vi "Get Records by Channels.vi"(6 "Channel List (All)":string, 8 "error in (no error)":errorcluster, 9 "Record Length (-1)":i32=-1, 10 "Record Start Index (0)":i32, 11 "Live Graph Plotter in":refnum<class "Live Graph Plotter.lvclass">) -> (0 "error out":errorcluster, 2 "Records By Channels":T1(array[cluster]), 3 "Live Graph Plotter out":refnum<class "Live Graph Plotter.lvclass">, 4 "Channel List":string)   [LabVIEW 2025, in "Live Graph Plotter.lvclass"]
uses:
  Live Graph Plotter.lvclass
  Live Graph Plotter.lvclass/Live Graph Plotter.ctl
  <vilib>/regexp/Match Regular Expression.xnode
  <vilib>/Analysis/NI_AALBase.lvlib
  26139874-d73b-468d-aa02-11bd5f3709a5.vi
  <vilib>/Analysis/1siggen.llb/Ramp Pattern by Delta.vi
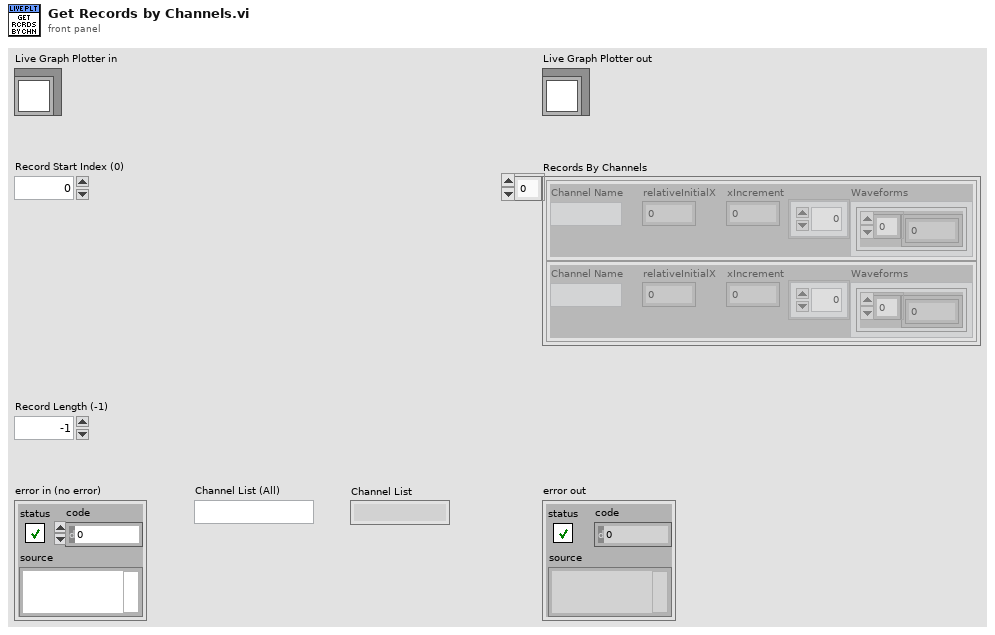
[diagram p1: front panel]
types:
  T1 = cluster{"Channel Name":string, "relativeInitialX":dbl, "xIncrement":dbl, "Waveforms":cluster{"wfm":dbl[]}[]}[]
  T2 = cluster{"Channel Name":string, "relativeInitialX":dbl, "xIncrement":dbl, "Waveforms":cluster{"wfm":dbl[]}[]}
  T3 = cluster{"relativeInitialX":dbl, "xIncrement":dbl, "wfm":dbl[]}[]
  T4 = cluster{"relativeInitialX":dbl, "xIncrement":dbl, "wfm":dbl[]}
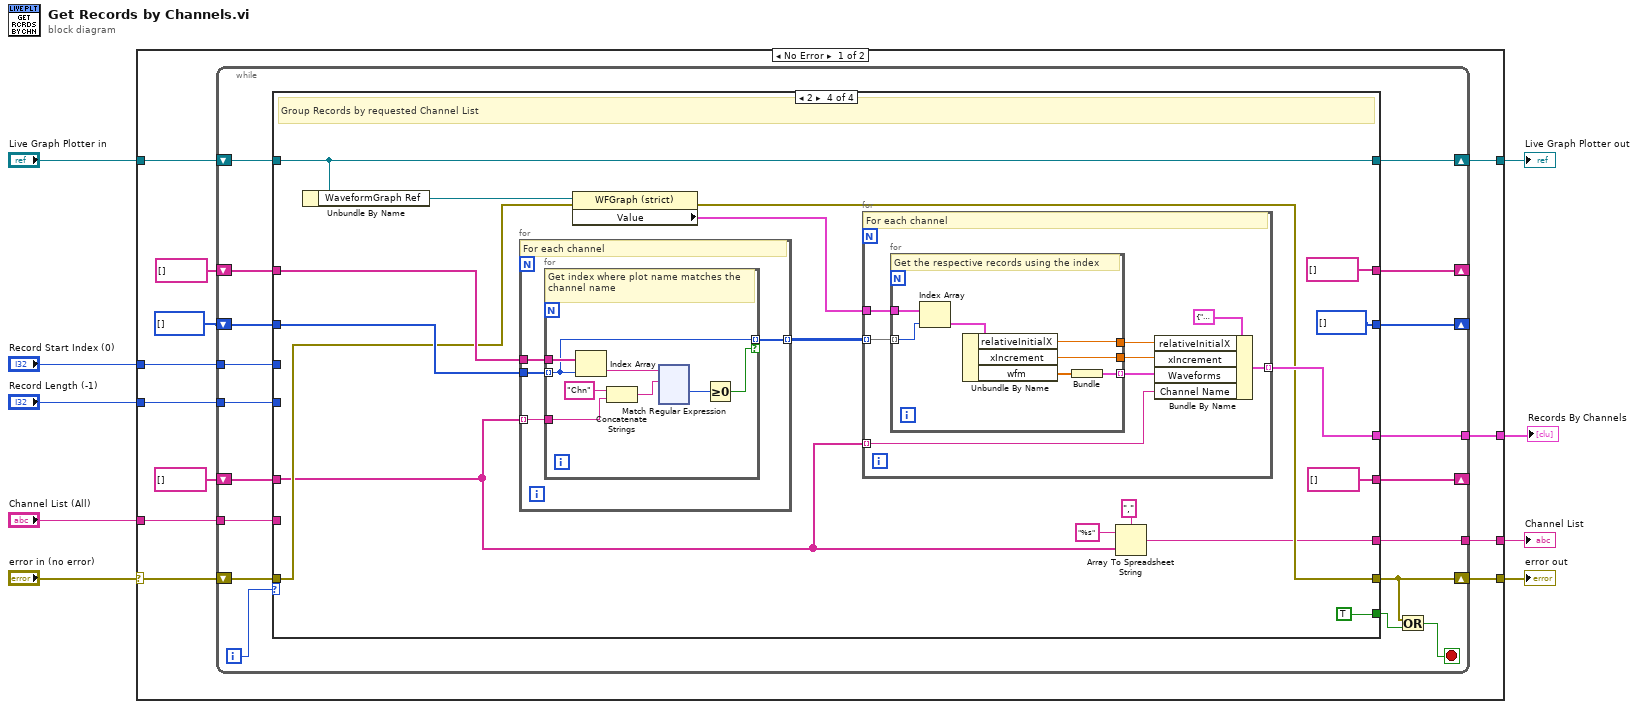
[diagram p0: block diagram]
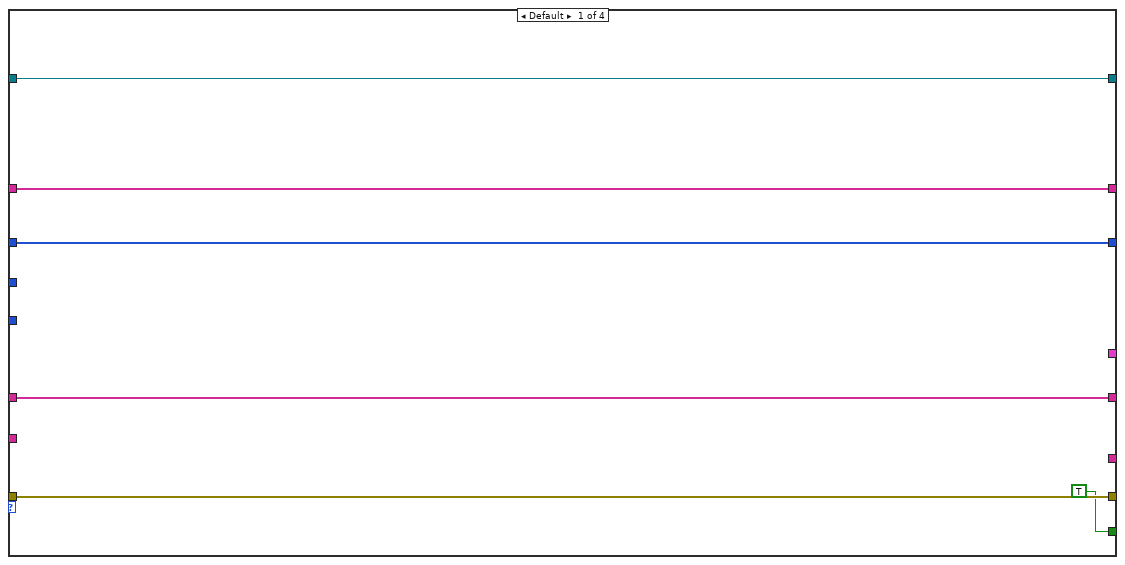
[diagram p2: hidden frame]
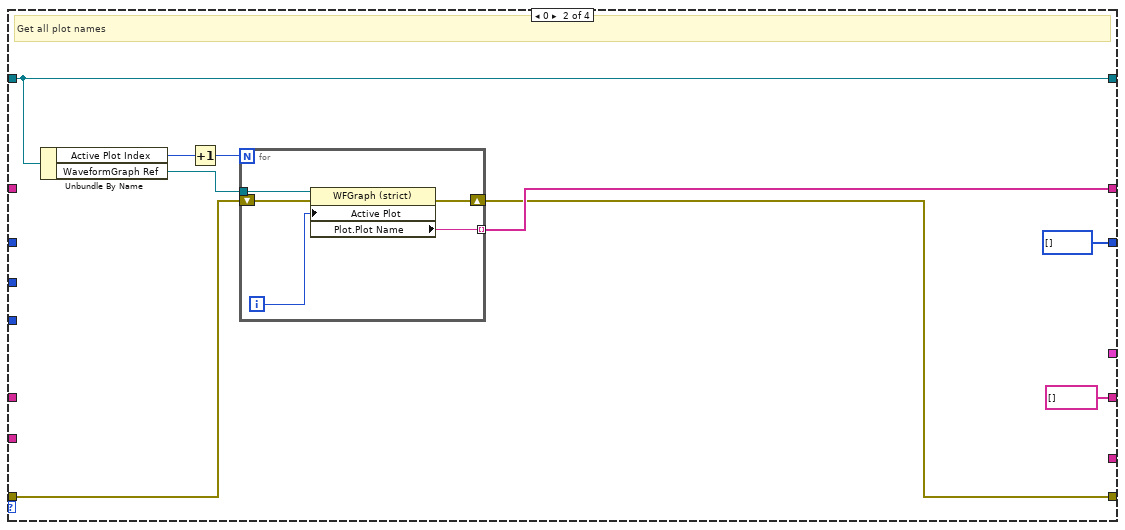
[diagram p3: hidden frame]
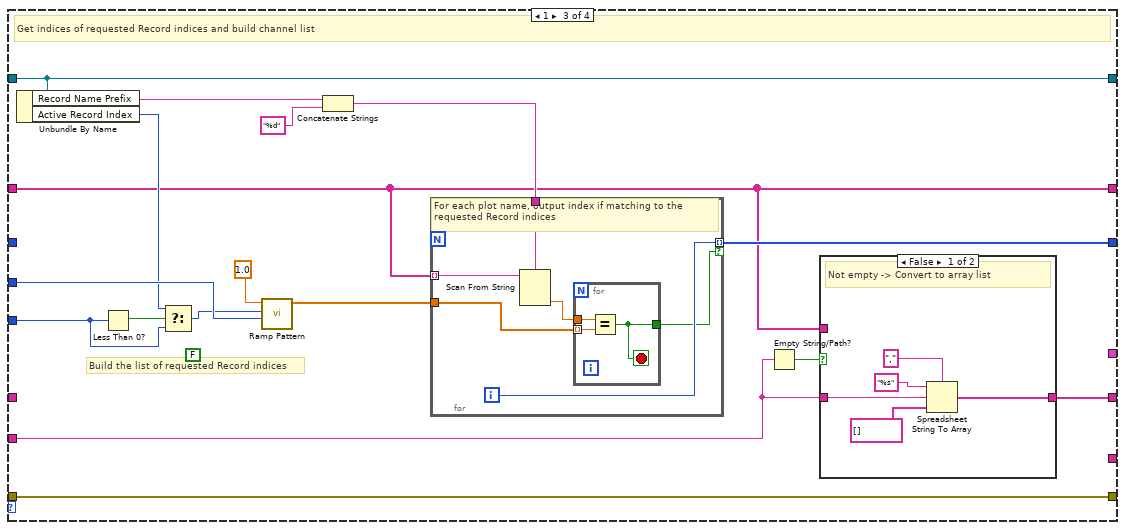
[diagram p4: hidden frame]
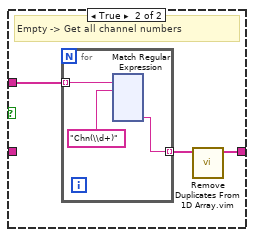
[diagram p5: hidden frame]
diagram:
  n1 = case shown="No Error" "error in (no error)" {
    selector: "error in (no error)" -> [w19 w379]
    tunnel: [w18 w379] -> w8
    tunnel: [w20 w378] -> w6
    tunnel: "Live Graph Plotter in" -> [w21 w378]
    tunnel: "Record Start Index (0)" -> [w16 _]
    tunnel: "Record Length (-1)" -> [w15 _]
    tunnel: "Channel List (All)" -> [w14 w377]
    tunnel: [w12 _] -> w2
    tunnel: [w10 w377] -> w1
    frame No Error {
      n2 = while {
        shift-right: [w35] -> w20
        shift-left: w21 -> [w39]
        shift-right: [w27] -> w18
        shift-left: w19 -> [w28]
        shift-right: [w37] -> _
        shift-left: string[] [] -> [w36]
        tunnel: w16 -> [w34]
        tunnel: w15 -> [w33]
        tunnel: w14 -> [w32]
        shift-right: [w31] -> _
        shift-left: i32[] [] -> [w30]
        tunnel: [w29] -> w12
        shift-right: [w24] -> _
        shift-left: string[] [] ("array type (2D Dbl)") -> [w23]
        tunnel: [w22] -> w10
        i -> [w38]
        stop <- w25 stop-if-true
        n3 = case shown="2" w38 {
          tunnel: w39 -> [w44 w54 w75 w230]
          tunnel: [w45 w51 w61 string[] []] -> w37
          tunnel: w36 -> [w45 _ w61 w232]
          tunnel: [w44 w54 w75 w230] -> w35
          tunnel: w34 -> [_ _ w76 _]
          tunnel: w33 -> [_ _ w73 _]
          tunnel: w32 -> [_ _ w63 _]
          tunnel: [w43 i32[] [] w69 i32[] []] -> w31
          tunnel: w30 -> [w43 _ _ w231]
          tunnel: [_ _ _ w226] -> w29
          tunnel: [w42 w48 w68 w223] -> w27
          tunnel: w28 -> [w42 w47 w68 w222]
          tunnel: [TRUE _ _ TRUE] -> w26
          tunnel: [w40 string[] [] ("array with duplicates removed") w60 string[] [] ("array with duplicates removed")] -> w24
          tunnel: w23 -> [w40 _ _ w219]
          tunnel: [_ _ _ w218] -> w22
          frame Default {
          }
          frame 0 {
            # "Get all plot names"
            n4 = Unbundle By Name(w54) -> ("Active Plot Index"=w53:i32, "WaveformGraph Ref"=w50:refnum<vi>)
            n5 = Increment(x=w53) -> (x+1=w52:i32)
            n6 = for {
              N: w52 -> [_]
              tunnel: w50 -> [w59]
              tunnel: [w57] -> w51 mode=indexing
              shift-right: [w56] -> w48
              shift-left: w47 -> [w55]
              i -> [w58]
              n7 = property class="WFGraph (strict)"(reference=w59, error in=w55, "Active Plot"=w58) -> (error out=w56:errorcluster, "Plot.Plot Name"=w57:string)  [unwired: 1 out]
            }
          }
          frame 1 {
            (unwired) FALSE ("exclude end?")
            # "Build the list of requested Record indices"
            # "Get indices of requested Record indices and build channel list"
            n8 = Unbundle By Name(w75) -> ("Record Name Prefix"=w67:string, "Active Record Index"=w72:i32)
            n9 = Less Than 0?(x=w73) -> (x < 0?=w74:bool)
            n10 = Select(t=w72, s=w74, f=w73) -> (s? t:f=w71:i32)
            n11 = call-poly <vilib>:"Ramp Pattern.vi"("start"=w76, "end"=w71, "delta"=1.0) -> ("Ramp Pattern"=w70:dbl[])  [unwired: 6 in, 2 out]
            n12 = Concatenate Strings(w67, "%d" ("format string")) -> (w65:string)
            n13 = for {
              tunnel: w61 -> [w212] mode=indexing
              tunnel: w70 -> [w207]
              tunnel: [w210] -> w69 mode=indexing if=w209
              tunnel: w65 -> [w208]
              i -> [w210]
              # "For each plot name, output index if matching to the requested Record indices"
              n14 = Scan From String(format string=w208, input string=w212) -> (output 1=w211:dbl)  [unwired: 3 in, 3 out]
              n15 = for {
                tunnel: w211 -> [w215]
                tunnel: w207 -> [w214] mode=indexing
                tunnel: [w213] -> w209
                stop <- w213 stop-if-true
                n16 = Equal?(x=w215, y=w214) -> (x = y?=w213:bool)
              }
            }
            n17 = Empty String/Path?(string/path=w63) -> (empty?=w62:bool)
            n18 = case shown="False" w62 {
              tunnel: w63 -> [w78 _]
              tunnel: w61 -> [_ w84]
              tunnel: [w77 w82] -> w60
              frame False {
                # "Not empty -> Convert to array list"
                n19 = Spreadsheet String To Array(delimiter (Tab)=",", format string="%s", spreadsheet string=w78, array type (2D Dbl)=string[] []) -> (array=w77:string[])
              }
              frame True {
                # "Empty -> Get all channel numbers"
                n20 = for {
                  tunnel: w84 -> [w86] mode=indexing
                  tunnel: [w85] -> w83 mode=indexing
                  n21 = xnode "Match Regular Expression"("input string"=w86, "regular expression"="Chn(\\d+)") -> ("submatch 1"=w85:string)  [unwired: 4 in, 5 out]
                }
                n22 = call "Remove Duplicates From 1D Array.vim"("array"=w83) -> ("array with duplicates removed"=w82:string[])  [unwired: 10 in]
              }
            }
          }
          frame 2 {
            # "Group Records by requested Channel List"
            n23 = Unbundle By Name(w230) -> ("WaveformGraph Ref"=w229:refnum<vi>)
            n24 = for {
              tunnel: w232 -> [w251]
              tunnel: w231 -> [w250]
              tunnel: w219 -> [w249] mode=indexing
              tunnel: [w248] -> w227 mode=indexing
              # "For each channel"
              n25 = for {
                tunnel: w251 -> [w259]
                tunnel: w250 -> [w253] mode=indexing
                tunnel: w249 -> [w255]
                tunnel: [w253] -> w248 mode=indexing if=w252
                # "Get index where plot name matches the channel name"
                n26 = Index Array(array=w259, index=w253) -> (element=w258:string)
                n27 = Concatenate Strings("Chn" ("regular expression"), w255) -> (w256:string)
                n28 = xnode "Match Regular Expression"("input string"=w258, "regular expression"=w256) -> ("offset past match"=w254:i32)  [unwired: 4 in, 4 out]
                n29 = Greater Or Equal To 0?(x=w254) -> (x >= 0?=w252:bool)
              }
            }
            n30 = property class="WFGraph (strict)"(reference=w229, error in=w222) -> (error out=w223:errorcluster, "Value"=w228:T3)  [unwired: 1 out]
            n31 = for {
              tunnel: w228 -> [w240]
              tunnel: w227 -> [w239] mode=indexing
              tunnel: w219 -> [w234] mode=indexing
              tunnel: [w233] -> w226 mode=indexing
              # "For each channel"
              n32 = for {
                tunnel: w240 -> [w247]
                tunnel: w239 -> [w246] mode=indexing
                tunnel: [w244] -> w235
                tunnel: [w243] -> w236
                tunnel: [w241] -> w237 mode=indexing
                # "Get the respective records using the index"
                n33 = Index Array(array=w247, index=w246) -> (element=w245:T4)
                n34 = Unbundle By Name(w245) -> ("relativeInitialX"=w244:dbl, "xIncrement"=w243:dbl, "wfm"=w242:dbl[])
                n35 = Bundle("wfm"=w242) -> (w241:cluster{"wfm":dbl[]})  [unwired: 1 in]
              }
              n36 = Bundle By Name(cluster=T2 {"Channel Name"="", "relativeInitialX"=0.0, "xIncrement"=0.0, "Waveforms"=[]}, "relativeInitialX"=w235, "xIncrement"=w236, "Waveforms"=w237, "Channel Name"=w234) -> (w233:T2)
            }
            n37 = Array To Spreadsheet String(delimiter (Tab)=",", array=w219, 3:"%s" ("format string")) -> (spreadsheet string=w218:string)
          }
        }
        n38 = Or(x=w27, y=w26) -> (x .or. y?=w25:bool)
      }
    }
    frame Error {
    }
  }
  "error out" <- w8
  "Live Graph Plotter out" <- w6
  "Records By Channels" <- w2
  "Channel List" <- w1
